vi "TomsToolsDocumentationTool_Global_OnCommand.vi"(10 "Command ID":string, 11 "Object":T1) -> ()   [LabVIEW 2015]
uses:
  Source Code/Model Messages/Load Project from Path Msg/Load Project from Path Msg.lvclass
  <resource>/Framework/Providers/API/ItemRef.ctl
panel:
  out "error out":errorcluster
  in  "error in":errorcluster
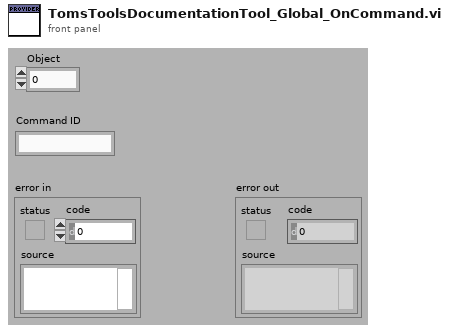
[diagram p1: front panel]
types:
  T1 = typedef "ItemRef.ctl" = u64
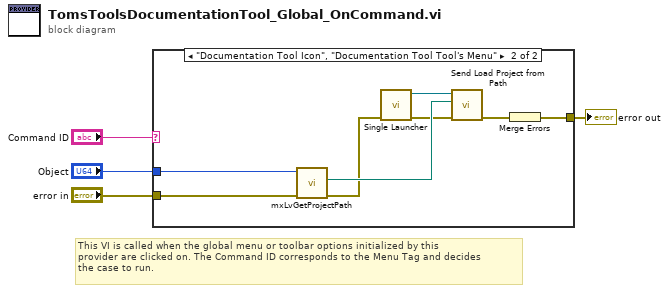
[diagram p0: block diagram]
diagram:
  # "This VI is called when the global menu or toolbar options initialized by this \nprovider are clicked on. The Command ID corresponds to the Menu Tag and decides\nthe case to run."
  n1 = case shown="\"Documentation Tool Icon\", \"Documentation Tool Tool's Menu\"" "Command ID" {
    tunnel: "error in" -> [w5 w7]
    tunnel: [w5 w13] -> w2
    tunnel: "Object" -> [_ w12]
    frame Default {
    }
    frame "Documentation Tool Icon", "Documentation Tool Tool's Menu" {
      n2 = call <resource>:"mxLvGetProjectPath.vi"("error in"=w7, "Item"=w12) -> ("error out"=w6:errorcluster, "Project Path"=w11:path)  [unwired: 7 in, 1 out]
      n3 = call "Single Launcher.vi"("error in (no errors)"=w6) -> ("error out"=w8:errorcluster, "Documentation Tool Model"=w10:refnum<class "Message Enqueuer.lvclass">)  [unwired: 9 in]
      n4 = call "Send Load Project from Path.vi"("error in (no error)"=w8, "Project Path"=w11, "Message Enqueuer"=w10) -> ("error out"=w9:errorcluster)  [unwired: 7 in, 1 out]
      n5 = Merge Errors(w9) -> (w13:errorcluster)
    }
  }
  "error out" <- w2
